vi "Test Coffee Shop Add Customer Broadcast Name.vi"(8 "error in (no error)":errorcluster, 11 "Coffee Shop Test In":refnum<class "Coffee Shop Test.lvclass">) -> (0 "error out":errorcluster, 3 "Coffee Shop Test Out":refnum<class "Coffee Shop Test.lvclass">)   [LabVIEW 2020, in "Coffee Shop Test.lvclass"]
uses:
  Coffee Shop Test.lvclass
  C:/Program Files (x86)/National Instruments/LabVIEW 2020/vi.lib/Asteme/LUnit/Test Case.lvclass
  Coffee Shop/Coffee Shop.lvclass
  C:/Program Files (x86)/National Instruments/LabVIEW 2020/vi.lib/Asteme/Triarc Framework/Process/Process.lvclass
  <vilib>/Asteme/Triarc Framework/Process/Process.lvclass/Process.ctl
  <vilib>/Asteme/LUnit/Test Case.lvclass/Test Case.ctl
  <vilib>/Asteme/LUnit/LUnit Assertion Result.lvclass/LUnit Assertion Result.ctl
  <vilib>/Asteme/Triarc Framework Test Suite/Support/Execution timer.vi
  <vilib>/Asteme/Triarc Framework/Process/Private/SubVIs/Wait for finish.vi
  <vilib>/Asteme/Triarc Framework/Process/Protected/Messaging/Enqueue Message.vi
  <vilib>/Asteme/Triarc Framework/Process/Private/SubVIs/Set Lifecycle State.vi
  <vilib>/Asteme/Triarc Framework/Process/Public/Lifecycle/Get Lifecycle State.vi
  <vilib>/Asteme/LUnit/Palette/Pass.vi
  <vilib>/Asteme/LUnit/Palette/Fail.vi
  <vilib>/Asteme/LUnit/Variant to string.vi
  <vilib>/Asteme/LUnit/Set Assertion Type.vi
  <vilib>/Utility/error.llb/Clear Errors.vi
  <vilib>/Asteme/LUnit/Add test result.vi
  <vilib>/Asteme/LUnit/LUnit Write Passed.vi
  <vilib>/Asteme/LUnit/LUnit Get Test Case.vi
  <vilib>/Asteme/LUnit/Assertion Result/LUnit Get Test Name.vi
  <vilib>/Asteme/LUnit/LUnit Write Message.vi
  <vilib>/Asteme/LUnit/LUnit Write Description.vi
  <vilib>/Asteme/LUnit/LUnit Write Assertion Type.vi
  <vilib>/Asteme/LUnit/Read Test Case Name.vi
  <vilib>/Utility/error.llb/Error Cluster From Error Code.vi
  <vilib>/Asteme/Triarc Framework Test Suite/Support/Event Helpers/Dequeue Event Message.vi
  <vilib>/Utility/Data Type/Get Type Information.vi
  <vilib>/Utility/LVClass/Get LV Class Name.vi
  <vilib>/Asteme/LUnit/LUnit Assertion Result.lvclass
  <vilib>/Asteme/Triarc Framework/Process/Process.lvclass
  <vilib>/Asteme/Triarc Framework Test Suite/Support/Event Helpers/Event Helpers.lvlib
  <vilib>/Asteme/LUnit/Test Case.lvclass
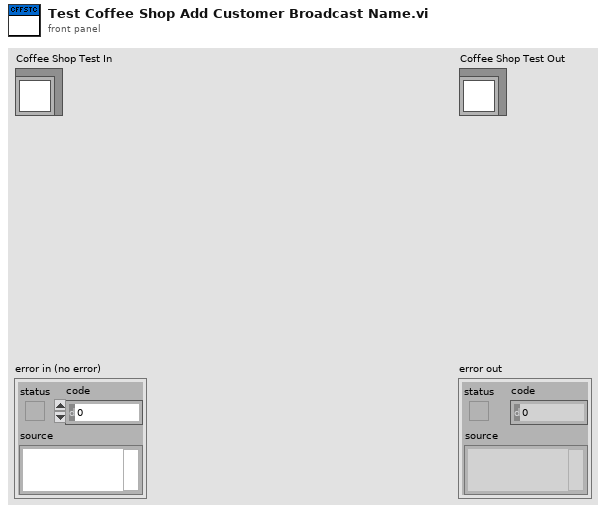
[diagram p1: front panel]
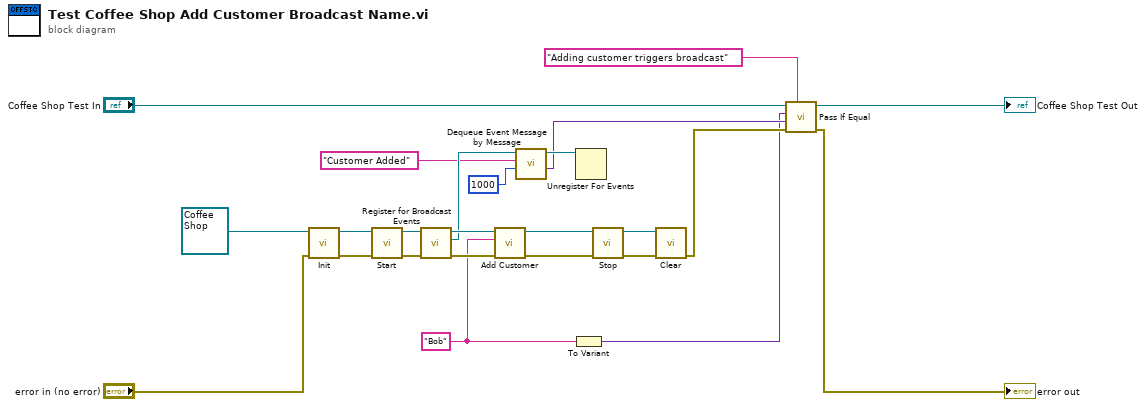
[diagram p0: block diagram]
diagram:
  w2 = "Bob" ("Name")
  n1 = call-dynamic "Init.vi"("error in (no error)"="error in (no error)", "Process In"=refnum<class "Coffee Shop.lvclass"> refnum ("Coffee Shop.lvclass")) -> ("error out"=w22:errorcluster, "Process Out"=w23:refnum<class "Coffee Shop.lvclass">)  [unwired: 8 in]
  n2 = call <vilib>:"Start.vi"("error in (no error)"=w22, "Process In"=w23) -> ("error out"=w21:errorcluster, "Process Out"=w14:refnum<class "Coffee Shop.lvclass">)  [unwired: 8 in]
  n3 = call <vilib>:"Register for Broadcast Events.vi"("error in (no error)"=w21, "Process In"=w14) -> ("error out"=w15:errorcluster, "Event Registration Refnum Out"=w12:refnum<event-registration>, "Process Out"=w13:refnum<class "Coffee Shop.lvclass">)  [unwired: 7 in]
  n4 = call "Add Customer.vi"("error in (no error)"=w15, "Name"=w2, "Coffee Shop in"=w13) -> ("error out"=w17:errorcluster, "Coffee Shop out"=w16:refnum<class "Coffee Shop.lvclass">)  [unwired: 7 in]
  n5 = call <vilib>:"Dequeue Event Message by Message.vi"("Timeout (-1)"=1000, "Message"="Customer Added", "Event Registration Refnum"=w12) -> ("Message Data"=w3:variant, "Event Registration Refnum Out"=w10:refnum<event-registration>)  [unwired: 4 in, 3 out]
  n6 = To Variant(anything=w2) -> (Variant=w1:variant)
  n7 = Unregister For Events(event registration refnum=w10) -> ()  [unwired: 1 in, 1 out]
  n8 = call <vilib>:"Stop.vi"("error in (no error)"=w17, "Process In"=w16) -> ("error out"=w19:errorcluster, "Process Out"=w20:refnum<class "Coffee Shop.lvclass">)  [unwired: 7 in, 1 out]
  n9 = call-dynamic "Clear.vi"("error in (no error)"=w19, "Application In"=w20) -> ("error out"=w6:errorcluster)  [unwired: 9 in]
  n10 = call <vilib>:"Pass If Equal.vi"("Description"="Adding customer triggers broadcast", "error in (no error)"=w6, "Actual"=w3, "Expected"=w1, "Test Case In"="Coffee Shop Test In") -> ("error out"=→"error out":errorcluster, "Test Case Out"=→"Coffee Shop Test Out":refnum<class "Coffee Shop Test.lvclass">)  [unwired: 5 in]
